vi "QuestionAsked.vi"(8 "Error In":errorcluster, 10 "Question":string, 11 "reference in":refnum<class "Clippy.lvclass">) -> (0 "Error Out":errorcluster, 3 "reference out":refnum<class "Clippy.lvclass">)   [LabVIEW 2020, in "Clippy.lvclass"]
uses:
  Clippy.lvclass
  AnimationTypes.ctl
  <vilib>/numeric/Random Number (Range) U64.vi
  <vilib>/numeric/sub_Random U32.vi
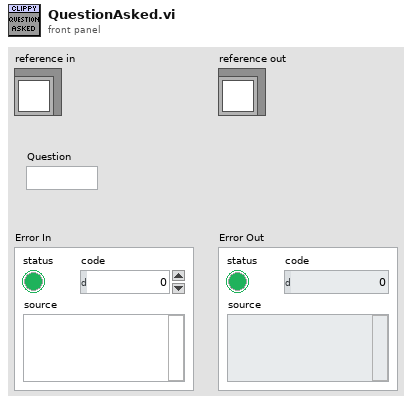
[diagram p1: front panel]
types:
  T1 = typedef "Clippy.lvclass/AnimationTypes.ctl" = enum16{"Congratulate", "LookRight", "SendMail", "Thinking", "Explain", "IdleRopePile", "IdleAtom", "Print", "Hide", "GetAttention", "Save", "GetTechy", "GestureUp", "Idle1_1", "Processing", "Alert", "LookUpRight", "IdleSideToSide", "GoodBye", "LookLeft", "IdleHeadScratch", "LookUpLeft", "CheckingSomething", "Hearing_1", "GetWizardy", "IdleFingerTap", "GestureLeft", "Wave", "GestureRight", "Writing", "IdleSnooze", "LookDownRight", "GetArtsy", "Show", "LookDown", "Searching", "EmptyTrash", "Greeting", "LookUp", "GestureDown", "RestPose", "IdleEyeBrowRaise", "LookDownLeft"}
  T2 = typedef "Clippy.lvclass/ObjectAttributes.ctl" = cluster{"ClippyPictureRef":refnum<vi>, "LastAnimation":T1, "LastAnimated":timestamp, "Visible":bool, "AnswerRef":refnum<vi>}
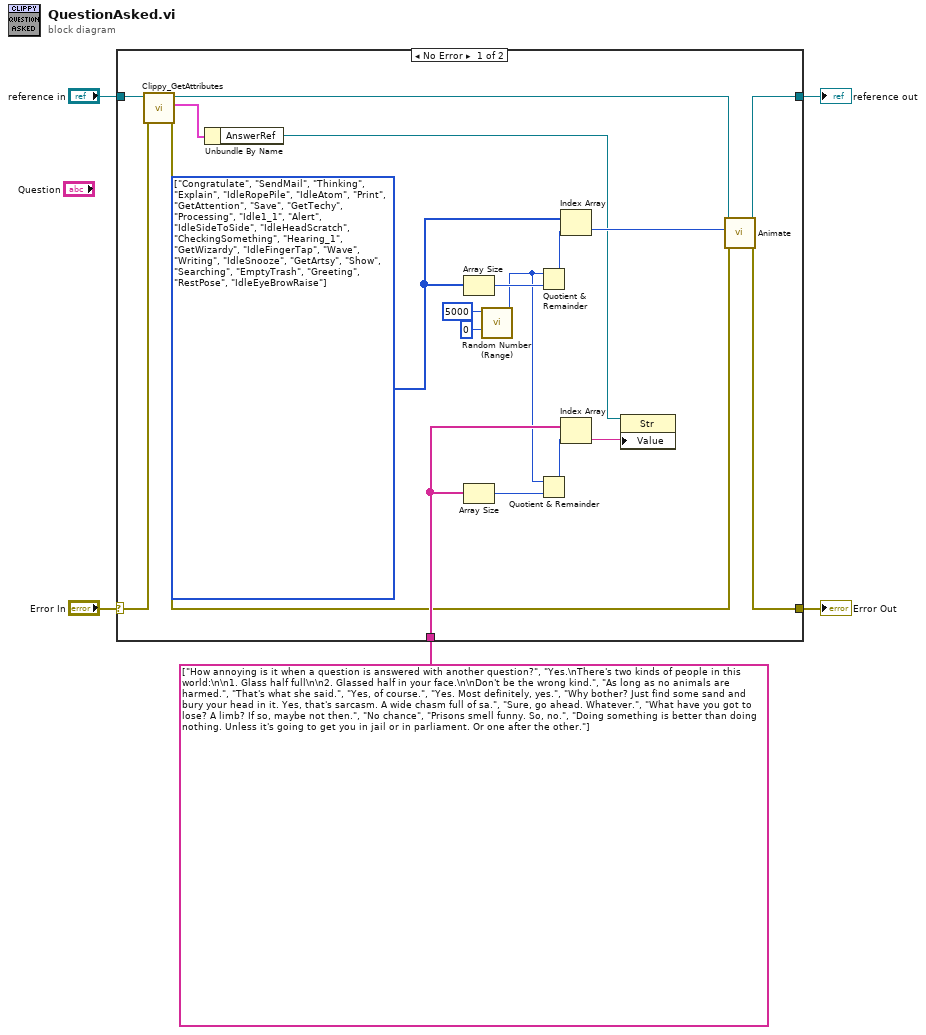
[diagram p0: block diagram]
diagram:
  n1 = case shown="No Error" "Error In" {
    selector: "Error In" -> [w24 w26]
    tunnel: [w6 w26] -> w4
    tunnel: [w14 w25] -> w2
    tunnel: "reference in" -> [w22 w25]
    tunnel: string[] ["How annoying is it when a question is answered with another question?", "Yes.\nThere's two kinds of people in this world:\n\n1. Glass half full\n\n2. Glassed half in your face.\n\nDon't be the wrong kind.", "As long as no animals are harmed.", "That's what she said.", "Yes, of course.", "Yes. Most definitely, yes.", "Why bother? Just find some sand and bury your head in it. Yes, that's sarcasm. A wide chasm full of sa.", "Sure, go ahead. Whatever.", "What have you got to lose? A limb? If so, maybe not then.", "No chance", "Prisons smell funny. So, no.", "Doing something is better than doing nothing. Unless it's going to get you in jail or in parliament. Or one after the other."] -> [w11 _]
    frame No Error {
      w18 = T1[] [enum."Congratulate", enum."SendMail", enum."Thinking", enum."Explain", enum."IdleRopePile", enum."IdleAtom", enum."Print", enum."GetAttention", enum."Save", enum."GetTechy", enum."Processing", enum."Idle1_1", enum."Alert", enum."IdleSideToSide", enum."IdleHeadScratch", enum."CheckingSomething", enum."Hearing_1", enum."GetWizardy", enum."IdleFingerTap", enum."Wave", enum."Writing", enum."IdleSnooze", enum."GetArtsy", enum."Show", enum."Searching", enum."EmptyTrash", enum."Greeting", enum."RestPose", enum."IdleEyeBrowRaise"] items=["Congratulate", "LookRight", "SendMail", "Thinking", "Explain", "IdleRopePile", "IdleAtom", "Print", "Hide", "GetAttention", "Save", "GetTechy", "GestureUp", "Idle1_1", "Processing", "Alert", "LookUpRight", "IdleSideToSide", "GoodBye", "LookLeft", "IdleHeadScratch", "LookUpLeft", "CheckingSomething", "Hearing_1", "GetWizardy", "IdleFingerTap", "GestureLeft", "Wave", "GestureRight", "Writing", "IdleSnooze", "LookDownRight", "GetArtsy", "Show", "LookDown", "Searching", "EmptyTrash", "Greeting", "LookUp", "GestureDown", "RestPose", "IdleEyeBrowRaise", "LookDownLeft"] ("Array")
      n2 = call "Clippy_GetAttributes.vi"("error in (no error)"=w24, "reference in"=w22) -> ("error out"=w7:errorcluster, "Data"=w23:T2, "reference out"=w15:refnum<class "Clippy.lvclass">)  [unwired: 6 in, 1 out]
      n3 = Unbundle By Name(w23) -> ("AnswerRef"=w9:refnum<vi>)
      n4 = Array Size(array=w18) -> (size(s)=w19:i32)
      n5 = Array Size(array=w11) -> (size(s)=w12:i32)
      n6 = call-poly <vilib>:"Random Number (Range).vi"("lower bound (0)"=u64 0, "upper bound (100)"=u64 5000) -> ("number"=w10:u64)  [unwired: 9 in]
      n7 = Quotient & Remainder(x=w10, y=w19) -> (x-y*floor(x/y)=w17:u64)  [unwired: 1 out]
      n8 = Quotient & Remainder(x=w10, y=w12) -> (x-y*floor(x/y)=w13:u64)  [unwired: 1 out]
      n9 = Index Array(array=w18, index=w17) -> (element=w16:T1)
      n10 = Index Array(array=w11, index=w13) -> (element=w8:string)
      n11 = property class="Str"(reference=w9, "Value"=w8) -> ()  [unwired: 1 in, 2 out]
      n12 = call-dynamic "Animate.vi"("Error In"=w7, "Animation"=w16, "reference in"=w15) -> ("Error Out"=w6:errorcluster, "reference out"=w14:refnum<class "Clippy.lvclass">)  [unwired: 7 in]
    }
    frame Error {
    }
  }
  "Error Out" <- w4
  "reference out" <- w2
